vi "KB-RS232-SendandReceiveMessage.vi"(8 "错误输入（无错误）":errorcluster, 9 "Timer":string, 10 "Command":string="*IDN?\n", 11 "VISA资源名称":refnum<visa-resource-name>) -> (0 "错误输出":errorcluster, 1 "响应":string, 2 "异常结果":bool, 3 "VISA资源名称输出":refnum<visa-resource-name>)   [LabVIEW 2015]
uses:
  C:/Program Files (x86)/National Instruments/LabVIEW 2015/examples/Instrument IO/Serial/support/Serial - Settings.ctl
  <vilib>/Instr/_visa.llb/VISA Configure Serial Port (Instr).vi
panel:
  out "长度":i32
  out "read buffer":string
  out "x/y":dbl
  in  "读取前延时(ms)":u32=100
  out "读取的字节":u32
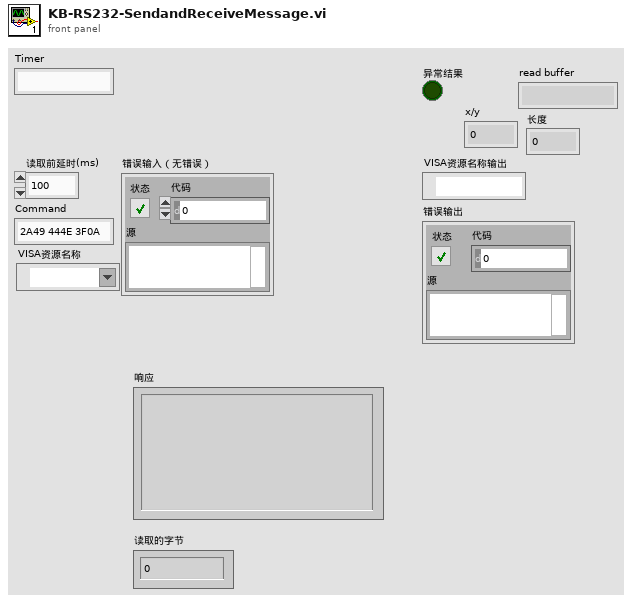
[diagram p1: front panel]
types:
  T1 = typedef "Serial - Settings.ctl" = cluster{"波特率":u32, "数据比特":u16, "奇偶":enum16{"None", "Odd", "Even", "Mark", "Space"}, "停止位":u16, "流控制":u16}
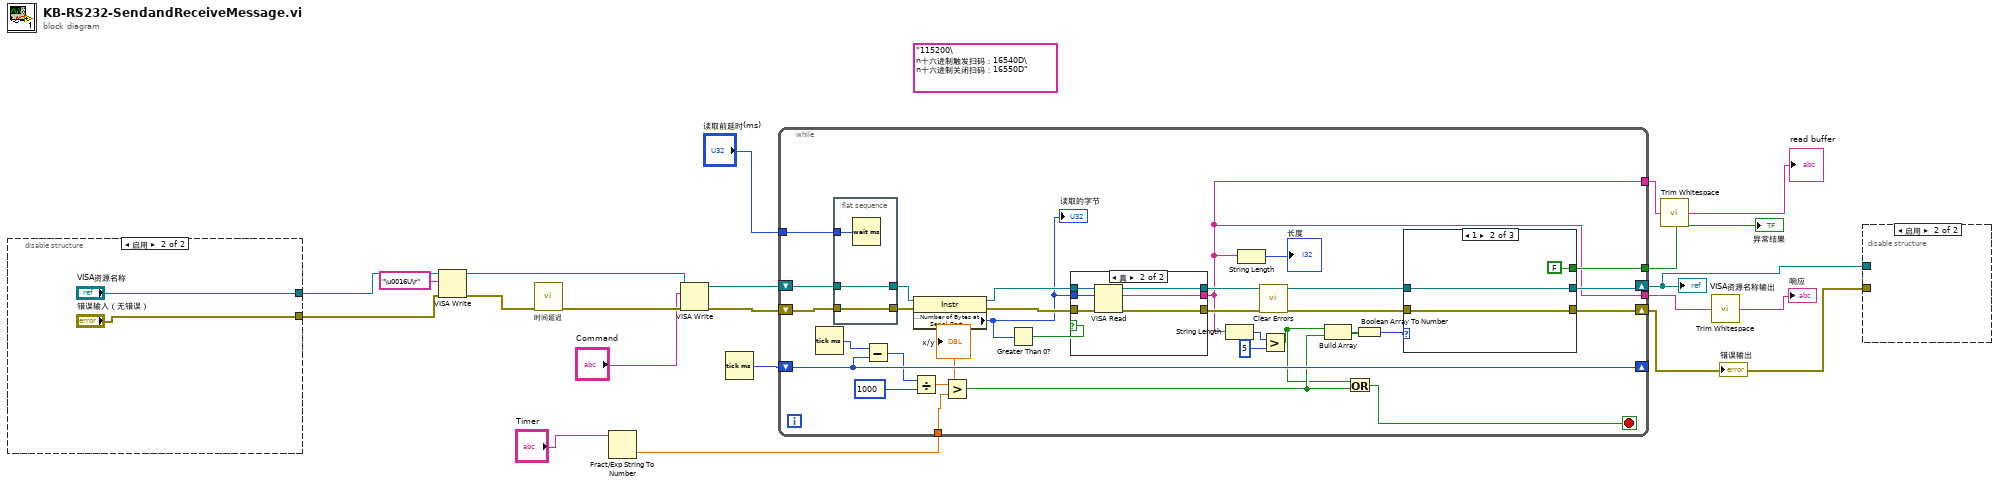
[diagram p0: block diagram]
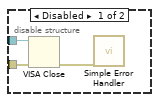
[diagram p2: hidden frame]
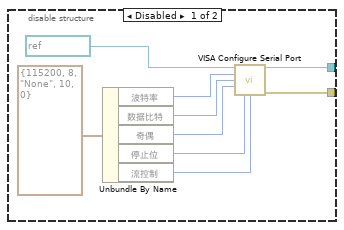
[diagram p3: hidden frame]
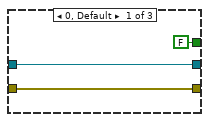
[diagram p4: hidden frame]
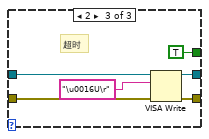
[diagram p5: hidden frame]
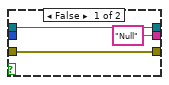
[diagram p6: hidden frame]
diagram:
  (unwired) "115200\n十六进制触发扫码：16540D\n十六进制关闭扫码：16550D"
  n1 = disable-structure shown="启用" {
    disable-tunnel: [w22 "VISA资源名称"] -> w13
    disable-tunnel: [w21 "错误输入（无错误）"] -> w12
    frame Disabled {
      n2 = Unbundle By Name(T1 {"波特率"=115200, "数据比特"=8, "奇偶"=enum."None", "停止位"=10, "流控制"=0} ("串口设置")) -> ("波特率"=w29:u32, "数据比特"=w28:u16, "奇偶"=w27:enum16{"None", "Odd", "Even", "Mark", "Space"}, "停止位"=w26:u16, "流控制"=w25:u16)
      n3 = call-poly "VISA Configure Serial Port"("VISA resource name"=refnum<visa-resource-name> "COM4" ("VISA资源名称"), "baud rate (9600)"=w29, "data bits (8)"=w28, "parity (0:none)"=w27, "stop bits (10: 1 bit)"=w26, "flow control (0:none)"=w25) -> ("VISA resource name out"=w22:refnum<visa-resource-name>, "error out"=w21:errorcluster)  [unwired: 3 in, 5 out]
    }
    frame Enabled {
    }
  }
  n4 = VISA Write(VISA resource name=w13, write buffer="\u0016U\r" ("写入缓冲区"), error in (no error)=w12) -> (VISA resource name out=w11:refnum<visa-resource-name>, error out=w9:errorcluster)  [unwired: 1 out]
  n5 = call "时间延迟"("error in (no error)"=w9) -> ("error out"=w8:errorcluster)  [unwired: 10 in]
  n6 = Fract/Exp String To Number(string="Timer") -> (number=w6:dbl)  [unwired: 3 in, 1 out]
  n7 = VISA Write(VISA resource name=w11, write buffer="Command", error in (no error)=w8) -> (VISA resource name out=w19:refnum<visa-resource-name>, error out=w20:errorcluster)  [unwired: 1 out]
  n8 = Tick Count (ms)() -> (millisecond timer value=w17:u32)
  n9 = while {
    tunnel: [w33] -> w4
    tunnel: "读取前延时(ms)" -> [w55]
    shift-right: [w39] -> w14
    shift-left: w20 -> [w61]
    shift-right: [w41] -> w15
    shift-left: w19 -> [w59]
    shift-right: [w50] -> _
    shift-left: w17 -> [w50]
    tunnel: [w38] -> w16
    tunnel: [w33] -> w2
    tunnel: w6 -> [w32]
    stop <- w46 stop-if-true
    n10 = Tick Count (ms)() -> (millisecond timer value=w51:u32)
    n11 = flat-sequence {
      tunnel: w61 -> [w84]
      tunnel: [w84] -> w60
      tunnel: w59 -> [w83]
      tunnel: [w83] -> w58
      tunnel: w55 -> [w85]
      frame #0 {
        n12 = Wait (ms)(milliseconds to wait=w85) -> ()  [unwired: 1 out]
      }
    }
    n13 = Subtract(x=w51, y=w50) -> (x-y=w49:u32)
    n14 = Divide(x=w49, y=u32 1000) -> (x/y=w47:dbl)
    "x/y" <- w47
    n15 = property class="Instr"(reference=w58, error in=w60) -> (reference out=w57:refnum<visa-resource-name>, error out=w56:errorcluster, "Serial Settings:Number of Bytes at Serial Port"=w54:u32)
    "读取的字节" <- w54
    n16 = Greater?(x=w47, y=w32) -> (0:w45:bool)
    n17 = Greater Than 0?(x=w54) -> (x > 0?=w53:bool)
    n18 = case shown="真" w53 {
      tunnel: w57 -> [w76 w82]
      tunnel: w56 -> [w75 w81]
      tunnel: ["Null" ("read buffer") w80] -> w33
      tunnel: w54 -> [_ w79]
      tunnel: [w76 w78] -> w42
      tunnel: [w75 w77] -> w52
      frame False {
      }
      frame True {
        n19 = VISA Read(VISA resource name=w82, byte count=w79, error in (no error)=w81) -> (VISA resource name out=w78:refnum<visa-resource-name>, read buffer=w80:string, error out=w77:errorcluster)  [unwired: 1 out]
      }
    }
    n20 = String Length(string=w33) -> (length=w37:i32)
    n21 = String Length(string=w33) -> (length=→"长度":i32)
    n22 = call <vilib>:"Clear Errors.vi"("error in (no error)"=w52) -> ("error out"=w40:errorcluster)  [unwired: 5 in, 1 out]
    n23 = Greater?(x=w37, y=5) -> (0:w35:bool)
    n24 = Build Array(w35, w45) -> (w44:bool[])
    n25 = Or(x=w35, y=w45) -> (x .or. y?=w46:bool)
    n26 = Boolean Array To Number(Boolean array=w44) -> (number=w43:u32)
    n27 = case shown="1" w43 {
      tunnel: w42 -> [w64 w67 w72]
      tunnel: [w64 w67 w71] -> w41
      tunnel: w40 -> [w63 w66 w70]
      tunnel: [w63 w66 w69] -> w39
      tunnel: [FALSE FALSE TRUE] -> w38
      frame 0, Default {
      }
      frame 1 {
      }
      frame 2 {
        # "超时"
        n28 = VISA Write(VISA resource name=w72, write buffer="\u0016U\r" ("Command 2"), error in (no error)=w70) -> (VISA resource name out=w71:refnum<visa-resource-name>, error out=w69:errorcluster)  [unwired: 1 out]
      }
    }
  }
  "VISA资源名称输出" <- w15
  "错误输出" <- w14
  "异常结果" <- w16
  n29 = call <vilib>:"Trim Whitespace.vi"("string"=w2) -> ("trimmed string"=→"read buffer":string)  [unwired: 1 in]
  n30 = call <vilib>:"Trim Whitespace.vi"("string"=w4) -> ("trimmed string"=→"响应":string)  [unwired: 1 in]
  n31 = disable-structure shown="启用" {
    disable-tunnel: w15 -> [w87 _]
    disable-tunnel: w14 -> [w86 _]
    frame Disabled {
      n32 = VISA Close(VISA resource name=w87, error in (no error)=w86) -> (error out=w88:errorcluster)
      n33 = call <vilib>:"Simple Error Handler.vi"("error in (no error)"=w88) -> ()  [unwired: 1 in, 8 out]
    }
    frame Enabled {
    }
  }
